vi "ProvideFood.vi"() -> ()   [LabVIEW 2013]
doc: "Use this template to build a producer/consumer design pattern with events to produce queue items. Use this design pattern instead of the User Interface Event Handler pattern for user interfaces when you want to execute code asynchronously in response to an event without slowing the user interface responsiveness."
uses:
  ObservableQueueData.ctl
  Food.lvclass
  Observable.lvclass/ObserverRegister.ctl
  Observable.lvclass/Observable.lvclass
panel:
  in  "ObserverList":i32(listbox)
  out "要放幾碗飯?":i32
  in  "ProvideFood":bool
  # "我是愛心媽媽"
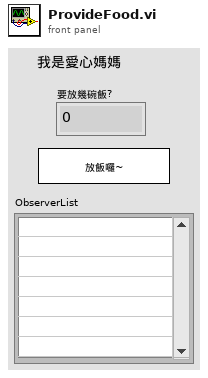
[diagram p1: front panel]
types:
  T1 = typedef "Observable.lvclass/ObserverRegister.ctl" = cluster{"Action":enum16{"Register", "UnRegister"}, "ObserverNotifierReference":refnum<notifier>}
  T2 = typedef "ObservableQueueData.ctl" = cluster{"ObservableAction":enum16{"Null", "Add/RemoveObserver", "NotifyObserver", "GetObserverList"}, "Variant":variant}
  T3 = enum16{"Null", "Add/RemoveObserver", "NotifyObserver", "GetObserverList"}
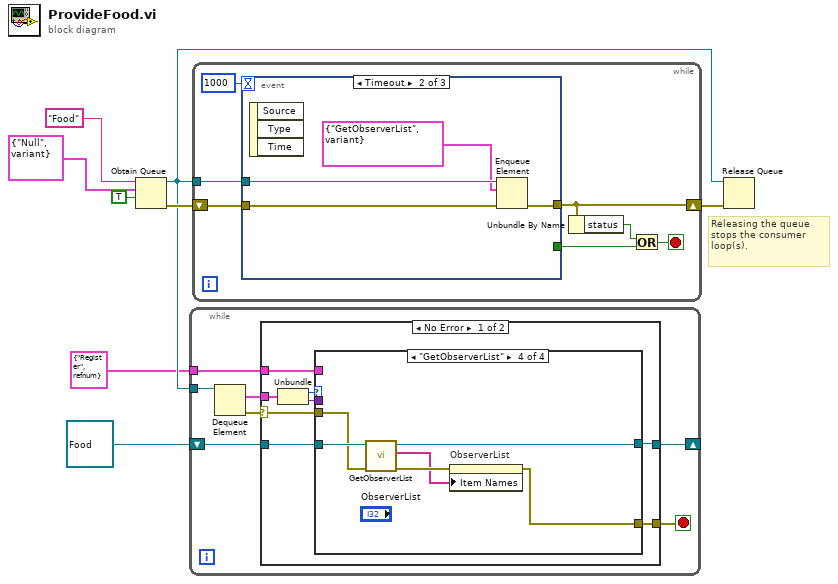
[diagram p0: block diagram]
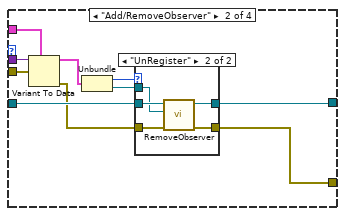
[diagram p3: hidden frame]
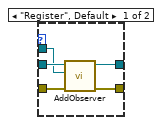
[diagram p4: hidden frame]
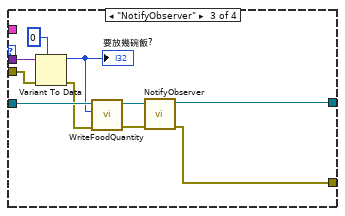
[diagram p5: hidden frame]
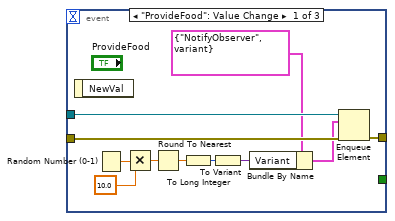
[diagram p7: hidden frame]
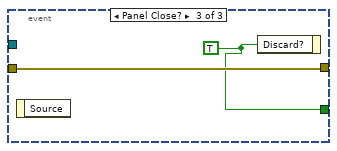
[diagram p8: hidden frame]
diagram:
  # "Releasing the queue stops the consumer loop(s)."
  n1 = Obtain Queue(name (unnamed)="Food", element data type=T2 {"ObservableAction"=enum."Null", "Variant"=variant} ("ObservableQueueData"), create if not found? (T)=TRUE) -> (queue out=w6:refnum<queue>, error out=w8:errorcluster)  [unwired: 2 in, 1 out]
  n2 = while {
    tunnel: w6 -> [w15]
    shift-right: [w10] -> _
    shift-left: refnum<class "Food.lvclass"> refnum ("Food.lvclass") -> [w11]
    tunnel: T1 {"Action"=enum."Register", "ObserverNotifierReference"=refnum} ("ObserverRegister") -> [w9]
    stop <- w12 stop-if-true
    n3 = Dequeue Element(queue=w15) -> (element=w13:T2, error out=w14:errorcluster)  [unwired: 2 in, 2 out]
    n4 = case shown="No Error" w14 {
      selector: w14 -> [w19 w63]
      tunnel: w13 -> [w23 _]
      tunnel: [w17 w63] -> w12
      tunnel: w11 -> [w20 w62]
      tunnel: [w18 w62] -> w10
      tunnel: w9 -> [w16 _]
      frame No Error {
        n5 = Unbundle(w23) -> ("ObservableAction"=w22:T3, "Variant"=w21:variant)
        n6 = case shown="\"GetObserverList\"" w22 {
          tunnel: w21 -> [_ w34 w55 _]
          tunnel: w20 -> [w25 w30 w52 w61]
          tunnel: w19 -> [w24 w35 w54 w60]
          tunnel: [w25 w28 w48 w59] -> w18
          tunnel: [w24 w26 w47 w56] -> w17
          tunnel: w16 -> [_ w33 _ _]
          frame "Null", Default {
          }
          frame "Add/RemoveObserver" {
            n7 = Variant To Data(error in=w35, type=w33, Variant=w34) -> (data=w32:T1, error out=w27:errorcluster)
            n8 = Unbundle(w32) -> ("Action"=w31:enum16{"Register", "UnRegister"}, "ObserverNotifierReference"=w29:refnum<notifier>)
            n9 = case shown="\"UnRegister\"" w31 {
              tunnel: w30 -> [w40 w45]
              tunnel: w29 -> [w38 w44]
              tunnel: [w39 w43] -> w28
              tunnel: w27 -> [w37 w42]
              tunnel: [w36 w41] -> w26
              frame "Register", Default {
                n10 = call-dynamic "AddObserver.vi"("error in (no error)"=w37, "ObserverNotifierReference"=w38, "Observable in"=w40) -> ("error out"=w36:errorcluster, "Observable out"=w39:refnum<class "Food.lvclass">)  [unwired: 7 in]
              }
              frame "UnRegister" {
                n11 = call-dynamic "RemoveObserver.vi"("error in (no error)"=w42, "ObserverNotifierReference"=w44, "Observable in"=w45) -> ("error out"=w41:errorcluster, "Observable out"=w43:refnum<class "Food.lvclass">)  [unwired: 7 in]
              }
            }
          }
          frame "NotifyObserver" {
            n12 = Variant To Data(error in=w54, type=0, Variant=w55) -> (data=w46:i32, error out=w51:errorcluster)
            "要放幾碗飯?" <- w46
            n13 = call-dynamic "WriteFoodQuantity.vi"("error in (no error)"=w51, "FoodQuantity"=w46, "Food in"=w52) -> ("error out"=w49:errorcluster, "Food out"=w50:refnum<class "Food.lvclass">)  [unwired: 7 in]
            n14 = call-dynamic "NotifyObserver.vi"("error in (no error)"=w49, "Food in"=w50) -> ("error out"=w47:errorcluster, "Food out"=w48:refnum<class "Food.lvclass">)  [unwired: 8 in]
          }
          frame "GetObserverList" {
            n15 = call-dynamic "GetObserverList.vi"("error in (no error)"=w60, "Observable in"=w61) -> ("error out"=w58:errorcluster, "ObserverClassName"=w57:string[], "Observable out"=w59:refnum<class "Food.lvclass">)  [unwired: 7 in]
            n16 = property on="ObserverList" class="LstBox (strict)"(error in=w58, "Item Names"=w57) -> (error out=w56:errorcluster)  [unwired: 1 in, 1 out]
          }
        }
      }
      frame Error {
        # "Return true in any case that should stop the loop."
      }
    }
  }
  n17 = while {
    shift-right: [w66] -> w7
    shift-left: w8 -> [w69]
    tunnel: w6 -> [w70]
    stop <- w67 stop-if-true
    n18 = event shown="[1] Timeout" {
      selector: _ -> [_ _ _]
      dyn-events: _ -> [_ _ _]
      timeout: 1000 -> [_ _ _]
      tunnel: w70 -> [w81 w85 _]
      tunnel: w69 -> [w80 w84 w87]
      tunnel: [w79 w82 w87] -> w66
      tunnel: [_ _ w86] -> w68
      event "ProvideFood": Value Change {
        n19 = event-data() -> ()  [unwired: 1 in, 1 out]
        n20 = Random Number (0-1)() -> (number: 0 to 1=w77:dbl)
        n21 = Multiply(x=w77, y=10.0) -> (x*y=w75:dbl)
        n22 = Round To Nearest(number=w75) -> (nearest integer value=w74:dbl)
        n23 = To Long Integer(number=w74) -> (32bit integer=w72:i32)
        n24 = To Variant(anything=w72) -> (Variant=w73:variant)
        n25 = Bundle By Name(cluster=T2 {"ObservableAction"=enum."NotifyObserver", "Variant"=variant} ("ObservableQueueData"), "Variant"=w73) -> (w71:T2)
        n26 = Enqueue Element(queue=w81, element=w71, error in (no error)=w80) -> (error out=w79:errorcluster)  [unwired: 1 in, 2 out]
      }
      event Timeout {
        n27 = event-data() -> ()  [unwired: 1 in, 3 out]
        n28 = Enqueue Element(queue=w85, element=T2 {"ObservableAction"=enum."GetObserverList", "Variant"=variant} ("ObservableQueueData"), error in (no error)=w84) -> (error out=w82:errorcluster)  [unwired: 1 in, 2 out]
      }
      event Panel Close? {
        w86 = TRUE ("stop")
        n29 = event-data() -> ()  [unwired: 1 in, 1 out]
        n30 = event-data("Discard?"=w86) -> ()  [unwired: 1 in, 1 out]
      }
    }
    n31 = Unbundle By Name(w66) -> ("status"=w65:bool)
    n32 = Or(x=w65, y=w68) -> (x .or. y?=w67:bool)
  }
  n33 = Release Queue(queue=w6, error in (no error)=w7) -> ()  [unwired: 1 in, 3 out]
